vi "Make GPS Basics.vi"(8 "Comms OK":bool, 9 "RMC":string) -> (2 "GPS Basics Out":T1 {"Course" format="%.2f"; "Speed" format="%.2f"; "Long" format="%.6f"; "Lat" format="%.6f"})   [LabVIEW 2015]
uses:
  GPS Basics.ctl
panel:
  in  "GPS Basics":T1 {"Course" format="%.2f"; "Speed" format="%.2f"; "Long" format="%.6f"; "Lat" format="%.6f"}
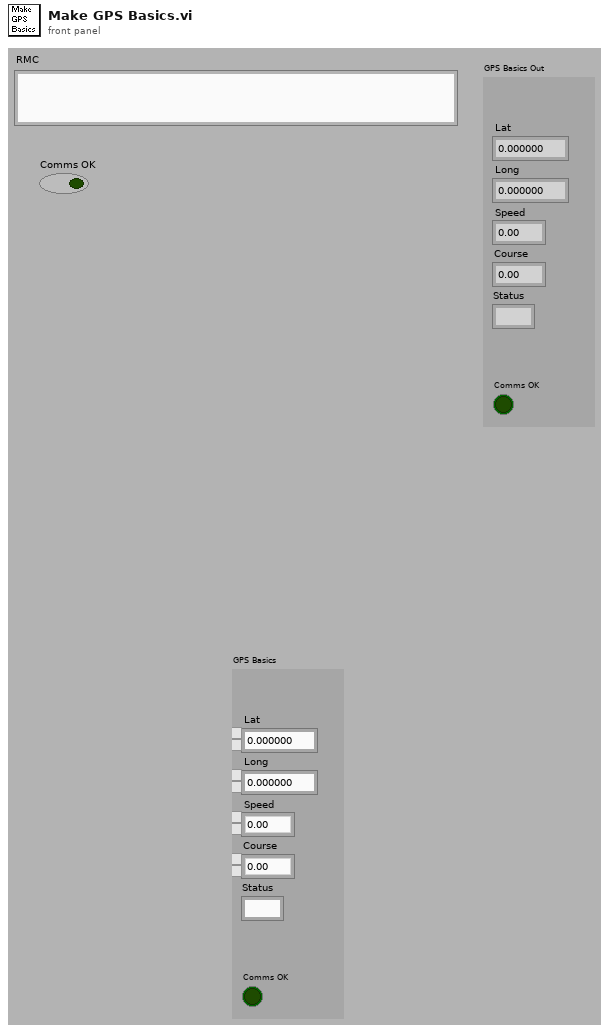
[diagram p1: front panel]
types:
  T1 = typedef "GPS Basics.ctl" = cluster{"Lat":dbl, "Long":dbl, "Speed":dbl, "Course":dbl, "Status":string, "Comms OK":bool}
  T2 = typedef "RMC.ctl" = cluster{"Time":string, "Status":string, "Lat":dbl, "Speed":dbl, "Course":dbl, "Long":dbl}
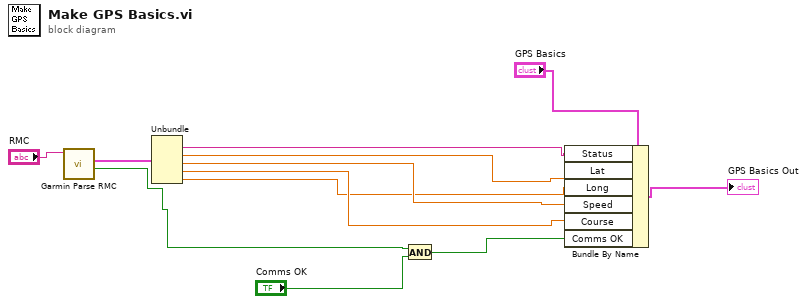
[diagram p0: block diagram]
diagram:
  n1 = call "Garmin Parse RMC.vi"("Input"="RMC") -> ("OK"=w3:bool, "RMC"=w9:T2)  [unwired: 6 in, 1 out]
  n2 = Unbundle(w9) -> ("Status"=w8:string, "Lat"=w7:dbl, "Speed"=w6:dbl, "Course"=w5:dbl, "Long"=w4:dbl)  [unwired: 1 out]
  n3 = And(x=w3, y="Comms OK") -> (x .and. y?=w1:bool)
  n4 = Bundle By Name(cluster="GPS Basics", "Status"=w8, "Lat"=w7, "Long"=w4, "Speed"=w6, "Course"=w5, "Comms OK"=w1) -> (→"GPS Basics Out":T1)
